vi "forma arreglo de números complejos.vi"(8 "Coeficientes de extinción":dbl[](array[slide]) scale=0.0..10.0, 11 "Índices de refracción":dbl[](array[slide]) scale=0.0..10.0) -> (3 "n + ik":cdb[](array[numeric]))   [LabVIEW 2013]
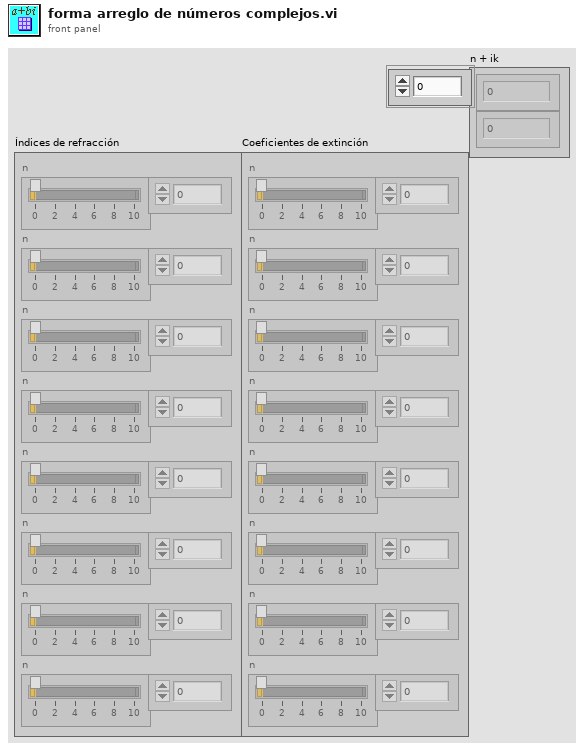
[diagram p1: front panel]
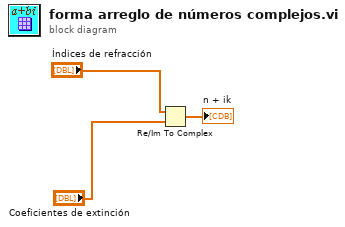
[diagram p0: block diagram]
diagram:
  n1 = Re/Im To Complex(1:"Coeficientes de extinción", 2:"Índices de refracción") -> (0:→"n + ik":cdb[])
